vi "GetThermAlarmStatusFlags.vi"(0 "VISA resource name":refnum<visa-resource-name>, 5 "error in":errorcluster) -> (14 "VISA resource name out":refnum<visa-resource-name>, 15 "Status Flags string":string, 16 "Status Flags":u8, 17 "Therm Alarm status flags":T1, 18 "Status Flags binary":string, 19 "error out":errorcluster)   [LabVIEW 2023, in "Thermotron 8800.lvlib"]
doc: "TALF\nCommand name: Send Therm Alarm status flags byte\nCommand type: System status\nDescription: The command allows you to retrieve the Therm Alarm status flags byte. The flags byte, a coded integer containing status about the Therm Alarm, is defined as follows:\nBits 0 through 7 \n1 High alarm \n2 Low alarm \n4 High warning \n8 Low warning \n16 Mute \n32 Over range \n64 Unused \n128 Open thermocouple\nSyntax: TALF?\nData type: Coded integer\nQuery example: TALF?\n8800 response: 17 (The Therm-Alarm status flags byte is mute and high alarm.)"
uses:
  Thermotron 8800.lvlib
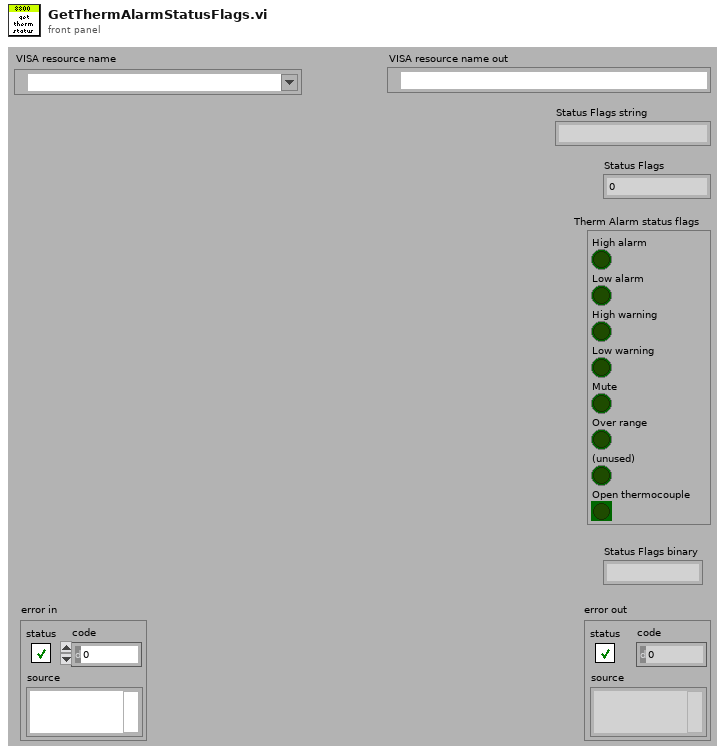
[diagram p1: front panel]
types:
  T1 = cluster{"High alarm":bool, "Low alarm":bool, "High warning":bool, "Low warning":bool, "Mute":bool, "Over range":bool, "(unused)":bool, "Open thermocouple":bool, "Open ":bool}
  T2 = cluster{"Boolean array[0]":bool, "Boolean array[1]":bool, "Boolean array[2]":bool, "Boolean array[3]":bool, "Boolean array[4]":bool, "Boolean array[5]":bool, "Boolean array[6]":bool, "Boolean array[7]":bool, "Boolean array[8]":bool}
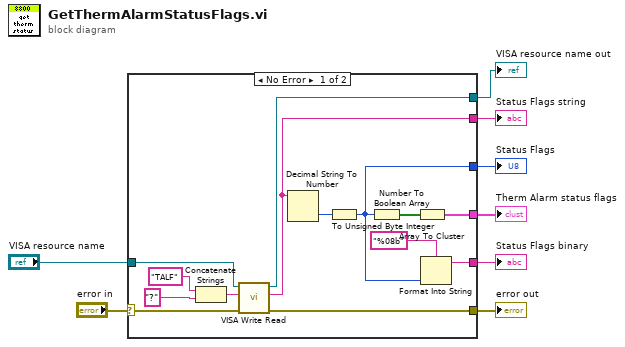
[diagram p0: block diagram]
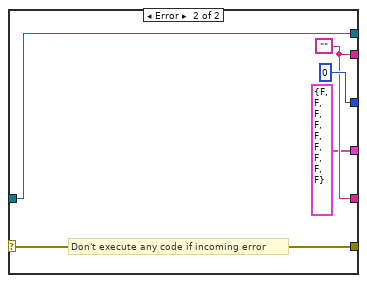
[diagram p2: hidden frame]
diagram:
  n1 = case shown="No Error" "error in" {
    selector: "error in" -> [w18 w25]
    tunnel: "VISA resource name" -> [w19 w27]
    tunnel: [w14 w25] -> w6
    tunnel: [w17 w27] -> w5
    tunnel: [w10 0] -> w4
    tunnel: [w11 w24] -> w1
    tunnel: [w9 w24] -> w3
    tunnel: [w15 T2 {"Boolean array[0]"=FALSE, "Boolean array[1]"=FALSE, "Boolean array[2]"=FALSE, "Boolean array[3]"=FALSE, "Boolean array[4]"=FALSE, "Boolean array[5]"=FALSE, "Boolean array[6]"=FALSE, "Boolean array[7]"=FALSE, "Boolean array[8]"=FALSE} ("Boolean array")] -> w2
    frame No Error {
      n2 = Concatenate Strings("TALF" ("string"), "?" ("string")) -> (w21:string)
      n3 = call "VISA Write Read.vi"("error in (no error)"=w18, "8800 Command"=w21, "VISA Refnum in"=w19) -> ("error out"=w14:errorcluster, "read buffer"=w9:string, "VISA Refnum out"=w17:refnum<visa-resource-name>)  [unwired: 6 in]
      n4 = Decimal String To Number(string=w9) -> (number=w13:i32)  [unwired: 2 in, 1 out]
      n5 = To Unsigned Byte Integer(number=w13) -> (unsigned 8bit integer=w10:u8)
      n6 = Number To Boolean Array(number=w10) -> (Boolean array=w16:bool[])
      n7 = Array To Cluster(array=w16) -> (cluster=w15:T2)
      n8 = Format Into String(format string="%08b", w10) -> (resulting string=w11:string)  [unwired: 2 in, 1 out]
    }
    frame Error {
      w24 = ""
      # "Don't execute any code if incoming error"
    }
  }
  "error out" <- w6
  "VISA resource name out" <- w5
  "Status Flags" <- w4
  "Status Flags string" <- w3
  "Therm Alarm status flags" <- w2
  "Status Flags binary" <- w1
